vi "Auto Loop 2.vi"(10 "auto #":u32, 11 "Call Context":T1) -> (0 "Loop 2 Value2":dbl, 1 "Loop 2 Value1":dbl, 2 "Loop 2 exit value":i32, 3 "Loop 2 SubState":T2=enum."auto")   [LabVIEW 2011]
uses:
  subStates.ctl
  <vilib>/Rock Robotics/WPI/DriverStation/WPI_DriverStationDerivedRobotMode.ctl
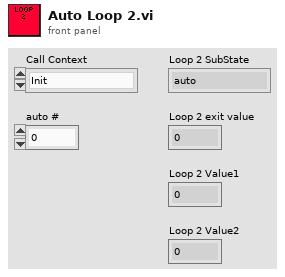
[diagram p1: front panel]
types:
  T1 = typedef "WPI_DriverStationDerivedRobotMode.ctl" = enum16{"Init", "Execute", "Stop"}
  T2 = typedef "subStates.ctl" = enum16{"null", "wait", "driver control", "auto", "manual override", "autoDrive", "hold position", "rotate", "end"}
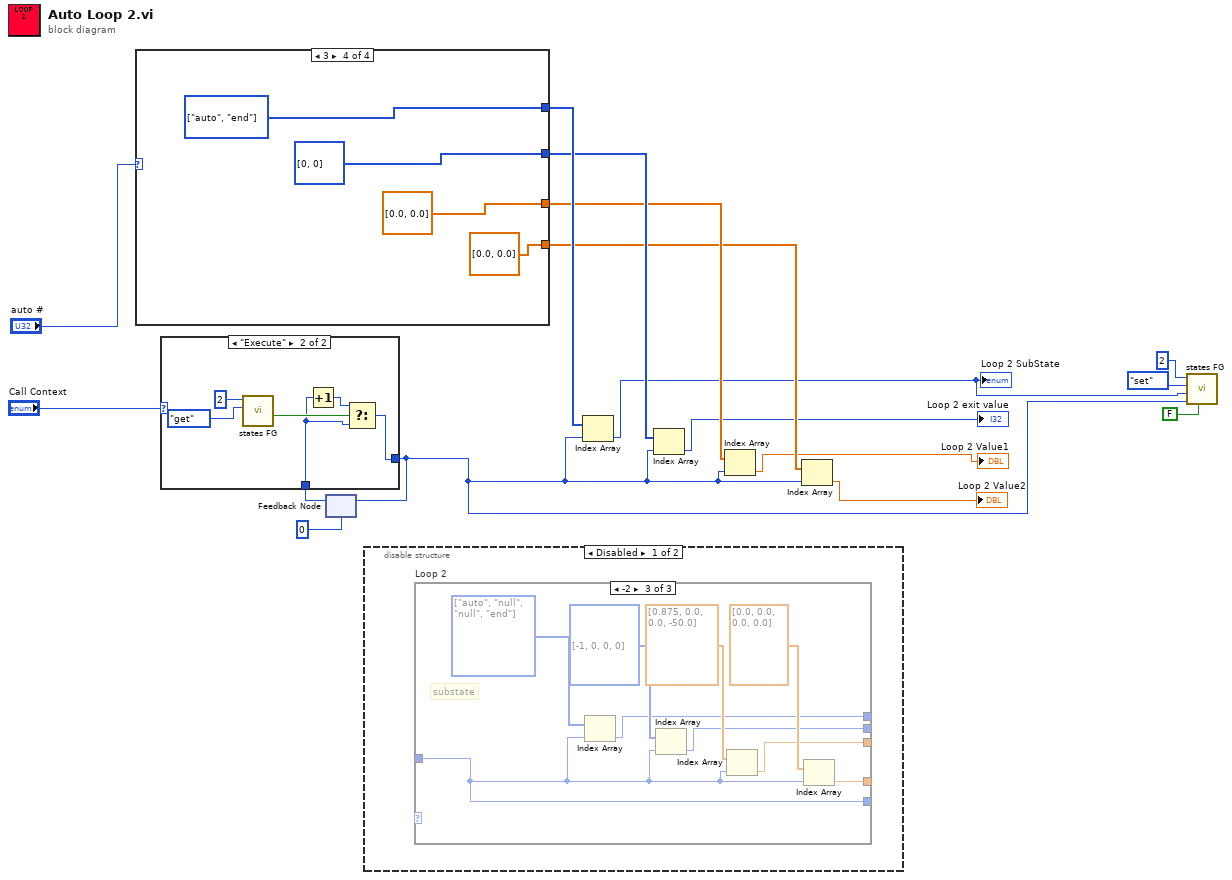
[diagram p0: block diagram]
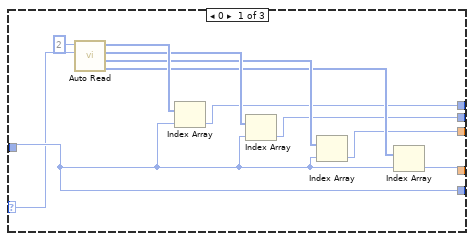
[diagram p2: hidden frame]
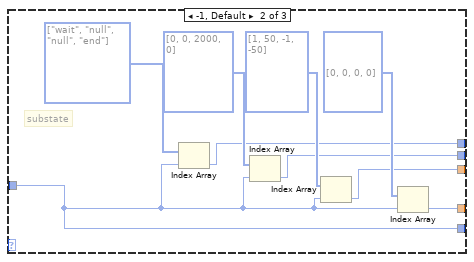
[diagram p3: hidden frame]
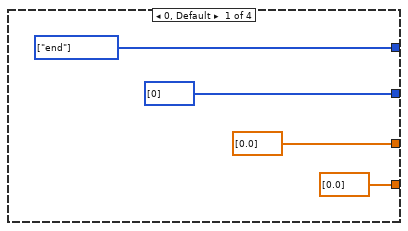
[diagram p5: hidden frame]
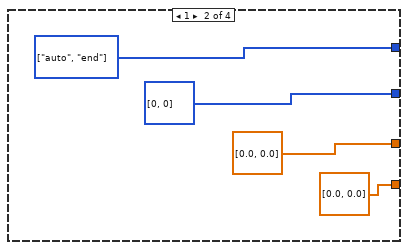
[diagram p6: hidden frame]
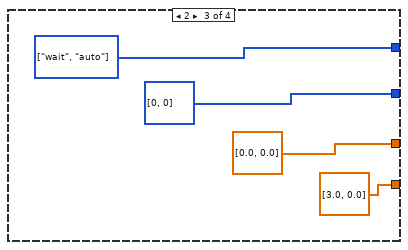
[diagram p7: hidden frame]
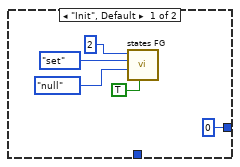
[diagram p8: hidden frame]
diagram:
  n1 = case shown="3" "auto #" {
    tunnel: [dbl[] [0.0] ("value2 array") dbl[] [0.0, 0.0] ("value2 array") dbl[] [3.0, 0.0] ("value2 array") dbl[] [0.0, 0.0] ("value2 array")] -> w8
    tunnel: [dbl[] [0.0] ("value1 array") dbl[] [0.0, 0.0] ("value1 array") dbl[] [0.0, 0.0] ("value1 array") dbl[] [0.0, 0.0] ("value1 array")] -> w9
    tunnel: [w18 w22 w26 w30] -> w11
    tunnel: [i32[] [0] ("exit value array") i32[] [0, 0] ("exit value array") i32[] [0, 0] ("exit value array") i32[] [0, 0] ("exit value array")] -> w10
    frame 0, Default {
      w18 = T2[] [enum."end"] items=["null", "wait", "driver control", "auto", "manual override", "autoDrive", "hold position", "rotate", "end"] ("substate array")
    }
    frame 1 {
      w22 = T2[] [enum."auto", enum."end"] items=["null", "wait", "driver control", "auto", "manual override", "autoDrive", "hold position", "rotate", "end"] ("substate array")
    }
    frame 2 {
      w26 = T2[] [enum."wait", enum."auto"] items=["null", "wait", "driver control", "auto", "manual override", "autoDrive", "hold position", "rotate", "end"] ("substate array")
    }
    frame 3 {
      w30 = T2[] [enum."auto", enum."end"] items=["null", "wait", "driver control", "auto", "manual override", "autoDrive", "hold position", "rotate", "end"] ("substate array")
    }
  }
  n2 = feedback #1(0 ("Value1 2")) -> (w13:i32)
  n3 = case shown="\"Execute\"" "Call Context" {
    tunnel: [0 ("Value1 2") w42] -> w2
    tunnel: w13 -> [_ w39]
    frame "Init", Default {
      n4 = call "states FG.vi"("exit in"=TRUE, "subState in"=subStates."null", "menu (get)"=enum16{"set", "get"}."set", "Loop ID"=2) -> ()  [unwired: 4 in, 4 out]
    }
    frame "Execute" {
      n5 = call "states FG.vi"("menu (get)"=enum16{"set", "get"}."get", "Loop ID"=2) -> ("exit out"=w41:bool)  [unwired: 6 in, 3 out]
      n6 = Increment(x=w39) -> (x+1=w43:i32)
      n7 = Select(t=w43, s=w41, f=w39) -> (s? t:f=w42:i32)
    }
  }
  n8 = feedback-in #1(w2) -> ()
  n9 = disable-structure shown="Disabled" {
    frame Disabled {
      n10 = case "Loop 2" shown="-2" {
        selector: _ -> [w44 _ _]
        tunnel: _ -> [w53 w55 w64]
        tunnel: [w48 w59 w68] -> _
        tunnel: [w47 w58 w67] -> _
        tunnel: [w46 w57 w66] -> _
        tunnel: [w45 w56 w65] -> _
        tunnel: [w53 w55 w64] -> _
        frame 0 {
          n11 = call "Auto Read.vi"("auto#"=w44, "loop #"=2) -> ("value 2s"=w49:i32[], "value 1s"=w50:i32[], "exit values"=w51:i32[], "substates"=w52:T2[])  [unwired: 6 in]
          n12 = Index Array(array=w52, index=w53) -> (element=w48:T2)
          n13 = Index Array(array=w51, index=w53) -> (element=w47:i32)
          n14 = Index Array(array=w50, index=w53) -> (element=w46:i32)
          n15 = Index Array(array=w49, index=w53) -> (element=w45:i32)
        }
        frame -1, Default {
          w63 = T2[] [enum."wait", enum."null", enum."null", enum."end"] items=["null", "wait", "driver control", "auto", "manual override", "autoDrive", "hold position", "rotate", "end"] ("SubState Array")
          # "val2"
          # "val1"
          # "exit"
          # "substate"
          n16 = Index Array(array=w63, index=w55) -> (element=w59:T2)
          n17 = Index Array(array=i32[] [0, 0, 2000, 0], index=w55) -> (element=w58:i32)
          n18 = Index Array(array=i32[] [1, 50, -1, -50], index=w55) -> (element=w57:i32)
          n19 = Index Array(array=i32[] [0, 0, 0, 0], index=w55) -> (element=w56:i32)
        }
        frame -2 {
          w72 = T2[] [enum."auto", enum."null", enum."null", enum."end"] items=["null", "wait", "driver control", "auto", "manual override", "autoDrive", "hold position", "rotate", "end"] ("SubState Array")
          # "val2"
          # "val1"
          # "exit"
          # "substate"
          n20 = Index Array(array=w72, index=w64) -> (element=w68:T2)
          n21 = Index Array(array=i32[] [-1, 0, 0, 0], index=w64) -> (element=w67:i32)
          n22 = Index Array(array=dbl[] [0.875, 0.0, 0.0, -50.0], index=w64) -> (element=w66:dbl)
          n23 = Index Array(array=dbl[] [0.0, 0.0, 0.0, 0.0], index=w64) -> (element=w65:dbl)
        }
      }
    }
    frame Enabled {
    }
  }
  n24 = Index Array(array=w11, index=w2) -> (element=w1:T2)
  "Loop 2 SubState" <- w1
  n25 = Index Array(array=w10, index=w2) -> (element=→"Loop 2 exit value":i32)
  n26 = Index Array(array=w9, index=w2) -> (element=→"Loop 2 Value1":dbl)
  n27 = Index Array(array=w8, index=w2) -> (element=→"Loop 2 Value2":dbl)
  n28 = call "states FG.vi"("exit in"=FALSE, "state # in"=w2, "subState in"=w1, "menu (get)"=enum16{"set", "get"}."set", "Loop ID"=2) -> ()  [unwired: 3 in, 4 out]
